vi "Calculate Remaining Processing Times.vi"(11 "Processing Times":u16[][](array[numeric])=[[34, 15, 38, 95], [2, 89, 19, 7], [54, 70, 28, 34], [61, 9, 87, 29]]) -> (3 "Remaining Processing Times":u16[][](array[numeric]))   [LabVIEW 2013, in "OSSP_Problem.lvclass"]
uses:
  OSSP_Problem.lvclass
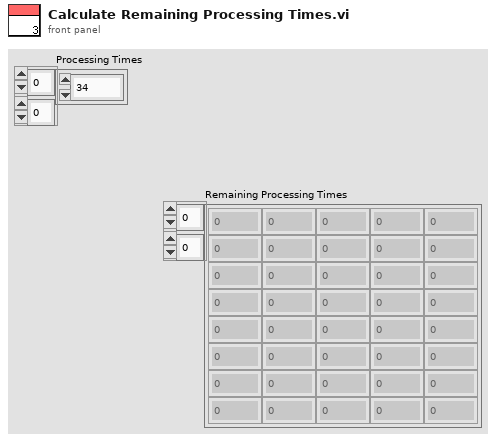
[diagram p1: front panel]
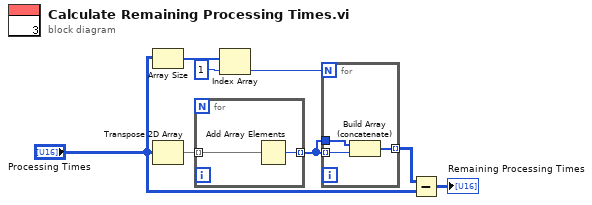
[diagram p0: block diagram]
diagram:
  n1 = Array Size(array="Processing Times") -> (size(s)=w7:i32[])
  n2 = Transpose 2D Array(2D array="Processing Times") -> (transposed array=w8:u16[][])
  n3 = for {
    tunnel: w8 -> [w10] mode=indexing
    tunnel: [w9] -> w4 mode=indexing
    n4 = Add Array Elements(numeric array=w10) -> (sum=w9:u16)
  }
  n5 = Index Array(array=w7, index=1) -> (element=w6:i32)
  n6 = for {
    N: w6 -> [_]
    tunnel: w4 -> [w12] mode=indexing
    tunnel: w4 -> [w13]
    tunnel: [w11] -> w3 mode=indexing
    n7 = Build Array (concatenate)(w13, w12) -> (w11:u16[])
  }
  n8 = Subtract(x=w3, y="Processing Times") -> (x-y=→"Remaining Processing Times":u16[][])
